vi "DDS_client_ring_text.vi"() -> ()   [LabVIEW 2012]
uses:
  <userlib>/LabRAD/internal/Build Packet SubVIs/Build Packet by Name.vi
  <userlib>/LabRAD/internal/Simple Request SubVIs/Simple Request by Name.vi
panel:
  in  "Amplitude (dBm)":dbl=-5.0
  in  "Frequency (MHz)":dbl=80.0
  in  "Channel":u16(ring) items=["global397", "866DP"]
  in  "update":bool
  out "client ID":u32
  out "welcome message":string
  in  "manager":T1={"address"="localhost", "port"=7682, "password"=""}
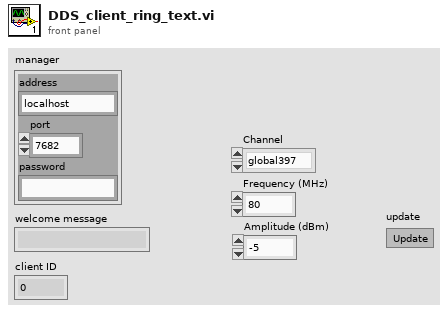
[diagram p1: front panel]
types:
  T1 = cluster{"address":string, "port":u16, "password":string}
  T2 = cluster{"RingText.Text":string, "Frequency (MHz)":dbl}
  T3 = cluster{"RingText.Text":string, "Amplitude (dBm)":dbl}
  T4 = cluster{"Setting":cluster{"ID":u32, "Name":string}, "Type Tag":string, "Data":string}[]
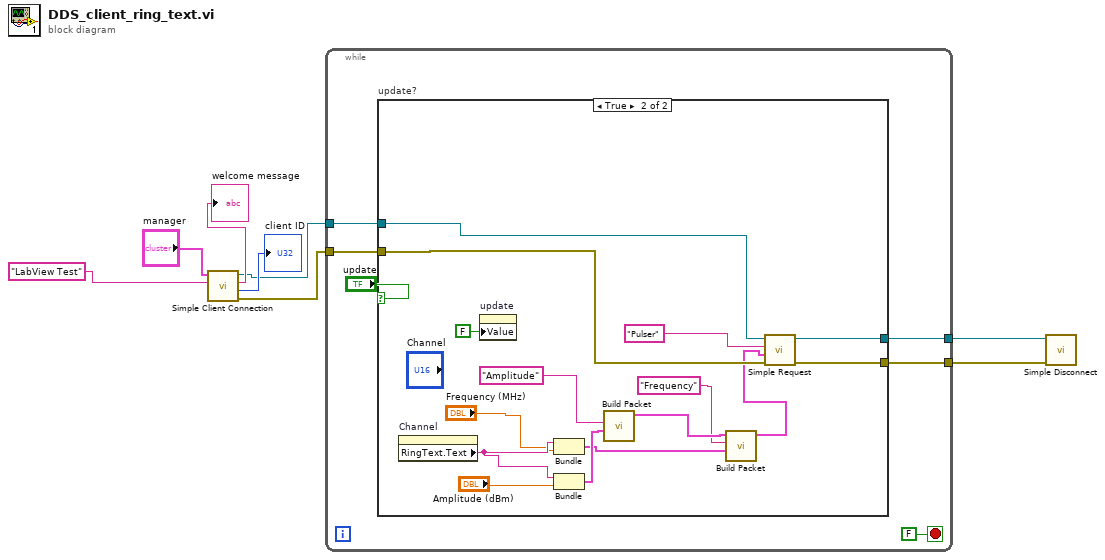
[diagram p0: block diagram]
diagram:
  n1 = call <userlib>:"Simple Client Connection.vi"("connection name (LabVIEW Client)"="LabView Test", "manager"="manager") -> ("error out"=w4:errorcluster, "client ID"=→"client ID":u32, "welcome message"=→"welcome message":string, "connection ID out"=w3:refnum<k5>)  [unwired: 2 in]
  n2 = while {
    tunnel: w4 -> [w12]
    tunnel: w3 -> [w11]
    tunnel: [w10] -> w2
    tunnel: [w9] -> w1
    stop <- FALSE stop-if-true
    n3 = case "update?" shown="True" "update" {
      tunnel: w12 -> [w15 w27]
      tunnel: w11 -> [w16 w28]
      tunnel: [w16 w26] -> w10
      tunnel: [w15 w25] -> w9
      frame False {
      }
      frame True {
        n4 = property on="Channel" class="Ring (strict)"() -> ("RingText.Text"=w18:string)  [unwired: 2 in, 2 out]
        n5 = property on="update" class="Bool (strict)"("Value"=FALSE ("update")) -> ()  [unwired: 2 in, 2 out]
        n6 = Bundle("RingText.Text"=w18, "Frequency (MHz)"="Frequency (MHz)") -> (w21:T2)  [unwired: 1 in]
        n7 = Bundle("RingText.Text"=w18, "Amplitude (dBm)"="Amplitude (dBm)") -> (w24:T3)  [unwired: 1 in]
        n8 = call-poly <userlib>:"Build Packet.vi"("data (empty)"=w24, "setting"="Amplitude") -> ("appended records"=w23:T4)  [unwired: 6 in, 2 out]
        n9 = call-poly <userlib>:"Build Packet.vi"("data (empty)"=w21, "setting"="Frequency", "records (empty)"=w23) -> ("appended records"=w22:T4)  [unwired: 5 in, 2 out]
        n10 = call-poly <userlib>:"Simple Request.vi"("error in (no error)"=w27, "records in (empty)"=w22, "target (Manager)"="Pulser", "connection ID"=w28) -> ("error out"=w25:errorcluster, "connection ID out"=w26:refnum<k5>)  [unwired: 2 in, 2 out]
      }
    }
  }
  n11 = call <userlib>:"Simple Disconnect.vi"("error in (no error)"=w1, "connection ID"=w2) -> ()  [unwired: 5 in, 1 out]
